vi "Control Fan.vi"(4 "error in (no error)":errorcluster, 7 "State Machine Data in":T1) -> (0 "error out":errorcluster, 3 "State Machine Data out":T1)   [LabVIEW 2015, in "Startup Processes.lvlib"]
uses:
  Startup Processes.lvlib
  _typedefs/State Machine Conditions.ctl
  _typedefs/Machine Modes.ctl
  _typedefs/Subpanel Names.ctl
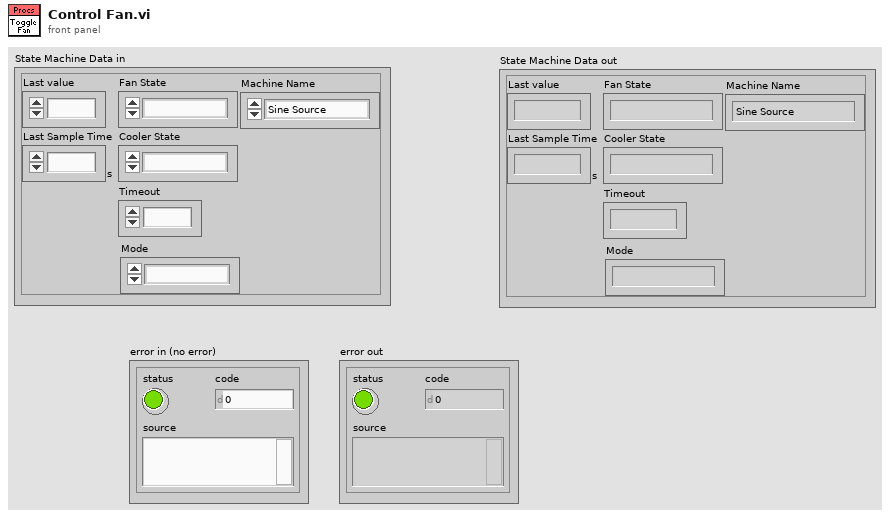
[diagram p1: front panel]
types:
  T1 = typedef "Startup Processes.lvlib/State Machine Conditions.ctl" = cluster{"Last value":dbl, "Last Sample Time":dbl[unit], "Fan State":enum16{"Off", "On"}, "Cooler State":enum16{"Off", "On"}, "Timeout":i32, "Mode":T2, "Machine Name":T3}
  T2 = typedef "Startup Processes.lvlib/Machine Modes.ctl" = enum16{"Startup", "Run"}
  T3 = typedef "Startup Processes.lvlib/Subpanel Names.ctl" = enum16{"Sine Source", "Ramp Source", "Hen House TC", "Dog House TC", "Out House TC"}
  T4 = enum16{"Write Fan State", "Write Cooler State", "Read"}
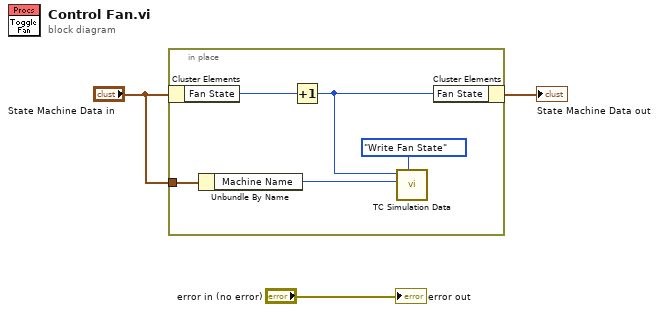
[diagram p0: block diagram]
diagram:
  n1 = in-place {
    in-place-border: "State Machine Data in" -> [w5]
    n2 = in-place-cluster #1("State Machine Data in") -> ("Fan State"=w8:enum16{"Off", "On"})
    n3 = Unbundle By Name(w5) -> ("Machine Name"=w4:T3)
    n4 = Increment(x=w8) -> (x+1=w6:enum16{"Off", "On"})
    n5 = call "TC Simulation Data.vi"("Function"=T4."Write Fan State", "Machine Name"=w4, "State In"=w6) -> ()  [unwired: 3 in, 3 out]
    n6 = in-place-cluster #1("Fan State"=w6) -> (→"State Machine Data out":T1)
  }
  "error out" <- "error in (no error)"
